vi "Test Sweep Mode vs Lockin_Vsg.vi"() -> ()   [LabVIEW 2019]
uses:
  src/Instrument.DAQ/Typedefs/Sweep.Configuration--Cluster.ctl
  src/Instrument.DAQ/Typedefs/Sweep.Channel--Cluster--Array.ctl
  src/Instrument.DAQ/Typedefs/Sweep.Channel--Cluster.ctl
  src/Instrument.DAQ/Typedefs/Sweep.Pattern--Enum.ctl
  src/Instrument.DAQ/Instrument.DAQ.lvclass
  <vilib>/measure/NI_MAPro.lvlib
  src/Instrument.Lockin/Instrument.Lockin.lvclass
  <vilib>/measure/maresamp.llb/Resample Waveform (single shot).vi
panel:
  in  "filename":string="100ms"
  in  "path":path=path "C:/user/patrick/hg/levy_inst_lockin/Tests/Test Sweep Mode/Test3"
  in  "OK":bool
  out "Sweep Mode (s)":u32=12
  out "LockinVsg (s)":u32=53
  in  "Configure Sweep":T1 {"Channels"."Table" format="%#_1f"; "Channels"."Channel" min=1 max=128; "Channels"."Start" format="%#_6p"; "Channels"."End" format="%#_6p"}
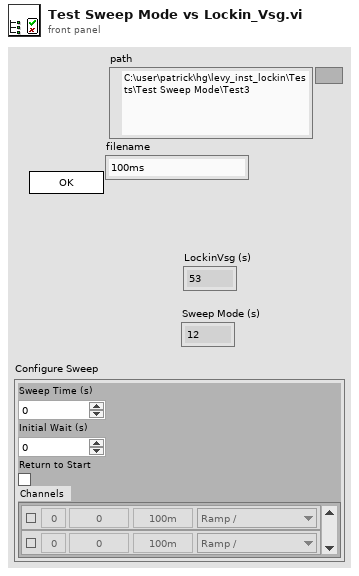
[diagram p1: front panel]
types:
  T1 = typedef "Instrument.Lockin.lvlib/Instrument.DAQ.lvclass/Sweep.Configuration--Cluster.ctl" = cluster{"Sweep Time (s)":dbl, "Initial Wait (s)":dbl, "Return to Start":bool, "Channels":T2}
  T2 = typedef "Instrument.Lockin.lvlib/Instrument.DAQ.lvclass/Sweep.Channel--Cluster--Array.ctl" = T3[]
  T3 = typedef "Instrument.Lockin.lvlib/Instrument.DAQ.lvclass/Sweep.Channel--Cluster.ctl" = cluster{"Enable?":bool, "Channel":u16, "Start":dbl, "End":dbl, "Pattern":T4, "Table":dbl[]}
  T4 = typedef "Instrument.Lockin.lvlib/Instrument.DAQ.lvclass/Sweep.Pattern--Enum.ctl" = enum16{"Ramp /", "Ramp /\\", "Smooth Ramp _/", "Smooth Ramp _/\\_", "Table"}
  T5 = enum32{"Invalid", "Standard", "Closed", "Hidden", "Minimized", "Maximized"}
  T6 = enum32{"invalid app kind", "Development System", "Run Time System", "Student Edition", "Embedded LabVIEW", "Evaluation", "Custom"}
  T7 = cluster{"Core":cluster{"Current VI Reference":refnum<vi>, "Close Panel on Exit?":bool}, "WFMs":waveform(dbl)[]}
  T8 = cluster{"Current VI Reference":refnum<vi>, "Close Panel on Exit?":bool}
  T9 = cluster{"Waveform Graph":dbl[], cluster{"key":string, "value":dbl}[]}
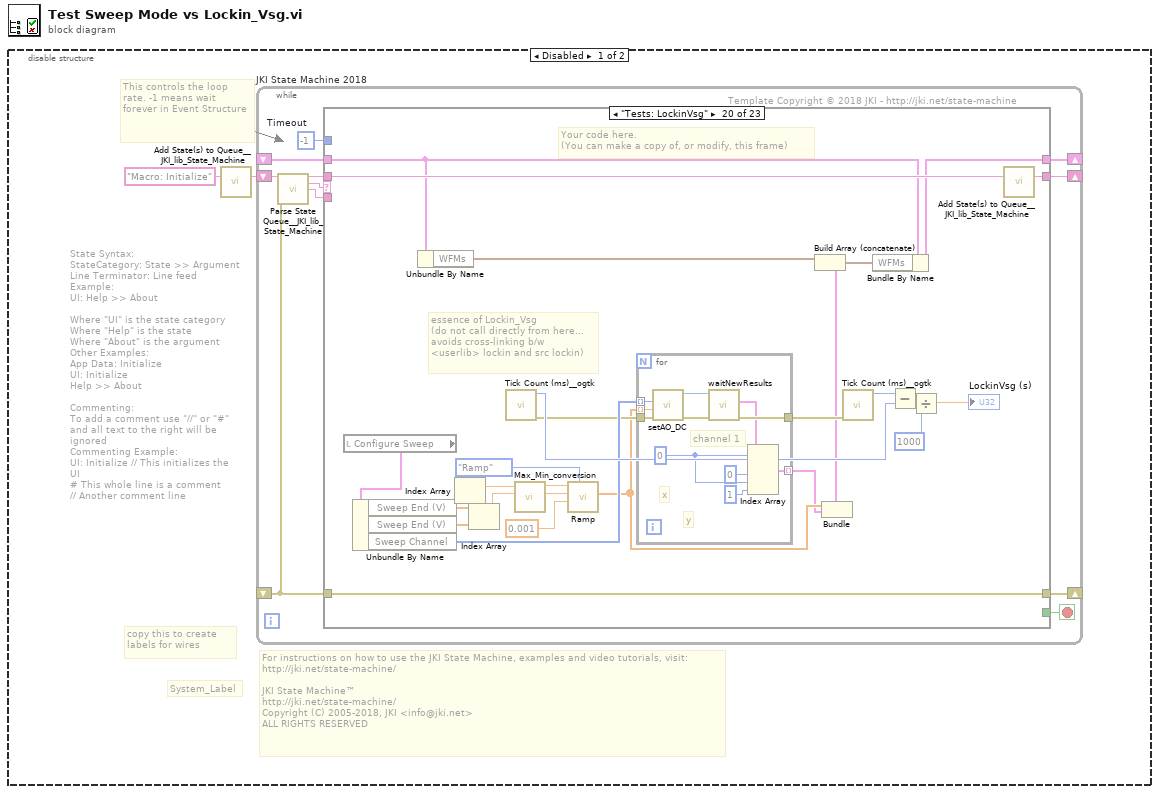
[diagram p0: block diagram]
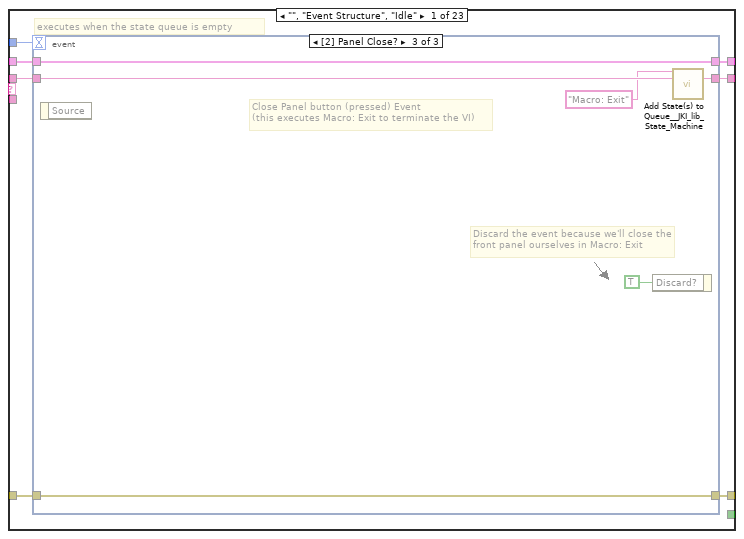
[diagram p2: hidden frame]
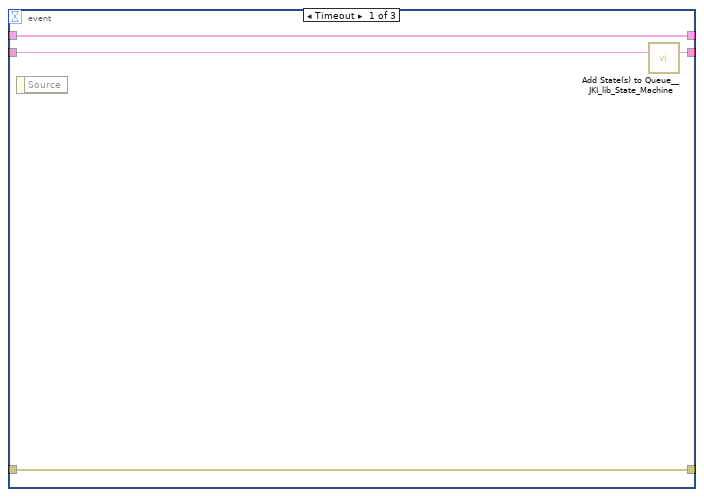
[diagram p3: hidden frame]
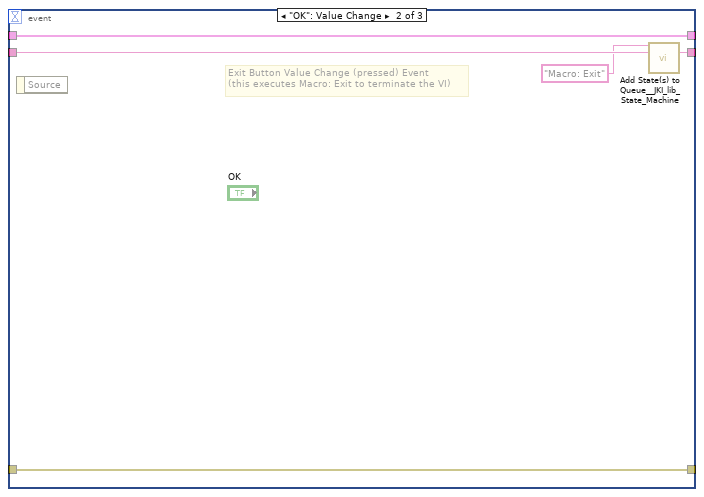
[diagram p4: hidden frame]
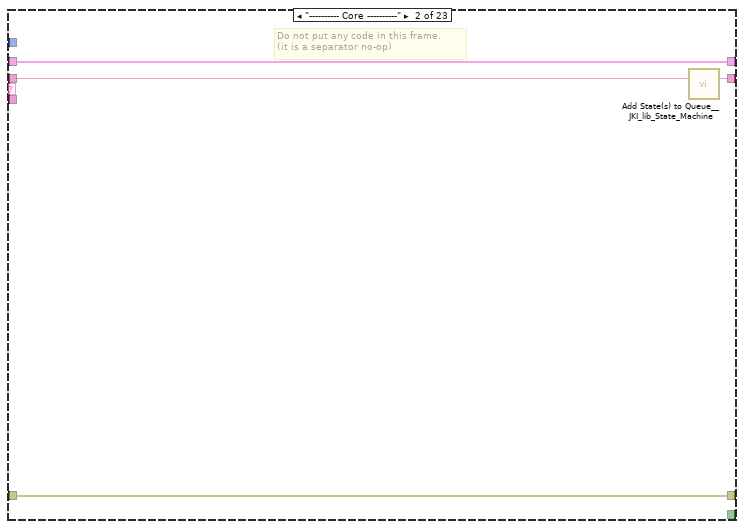
[diagram p5: hidden frame]
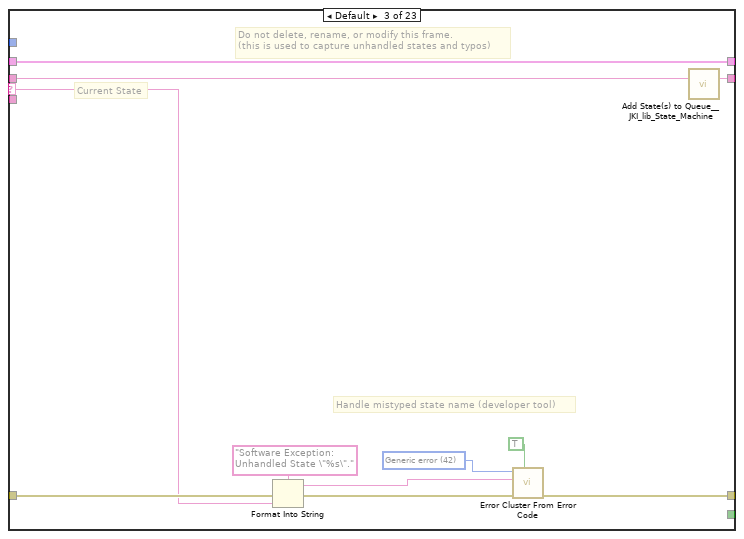
[diagram p6: hidden frame]
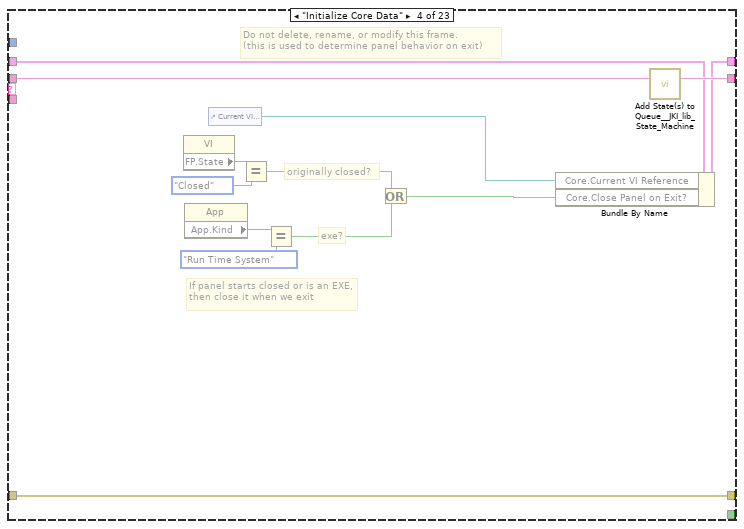
[diagram p7: hidden frame]
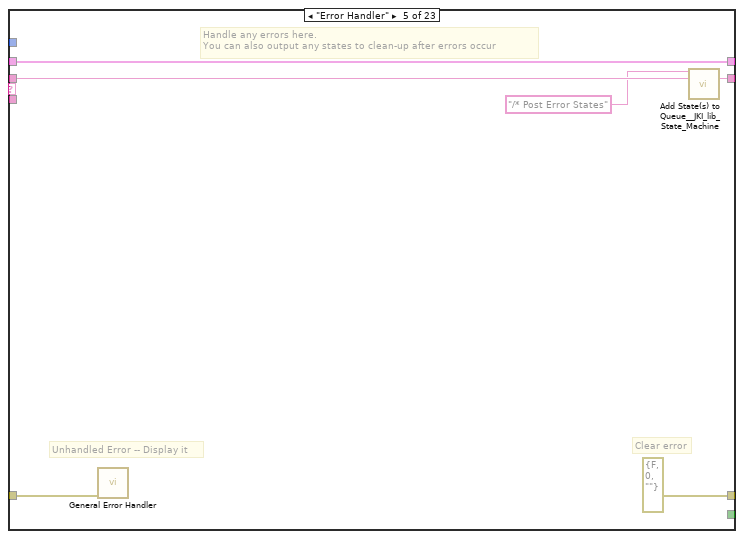
[diagram p8: hidden frame]
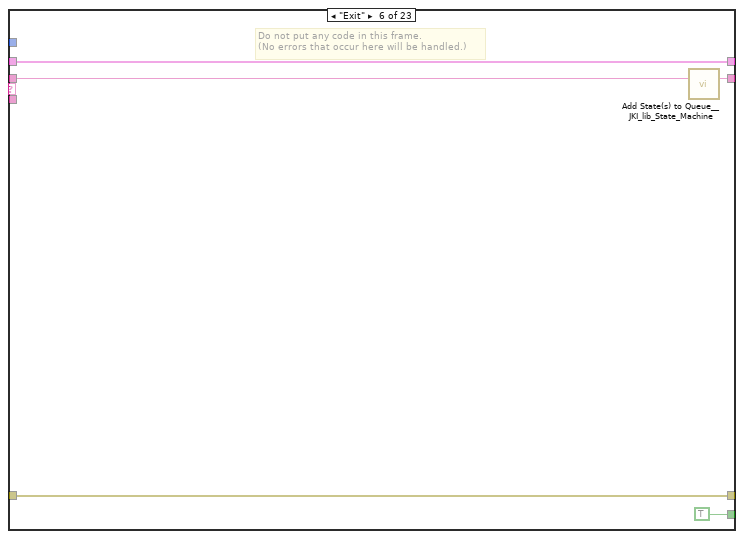
[diagram p9: hidden frame]
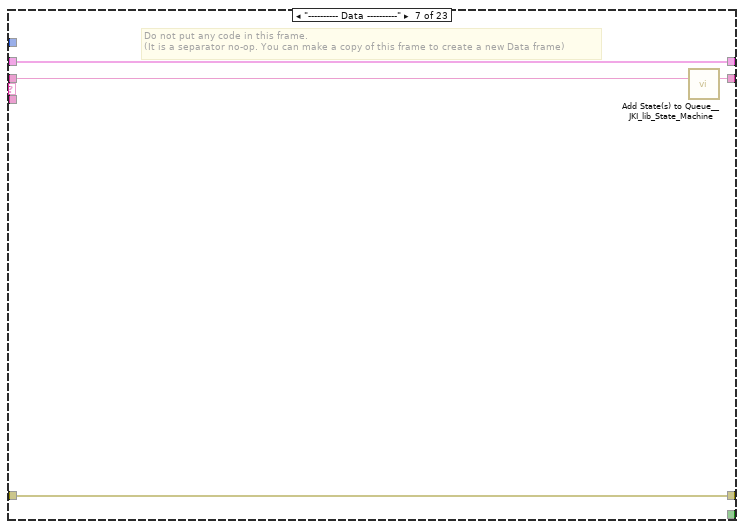
[diagram p10: hidden frame]
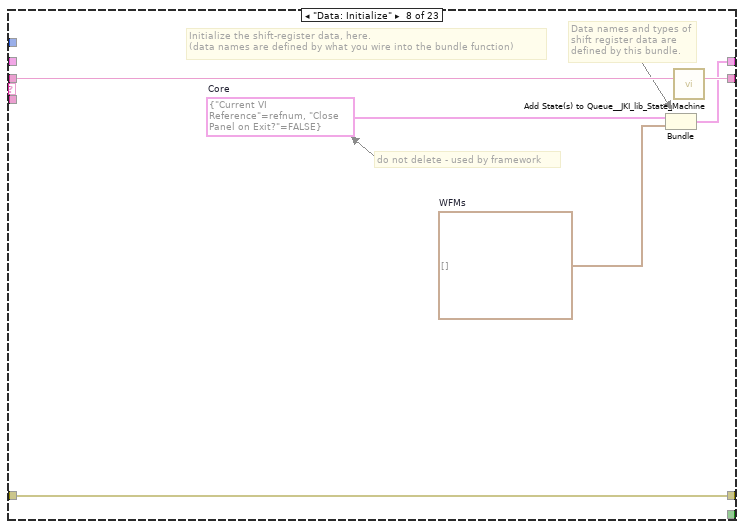
[diagram p11: hidden frame]
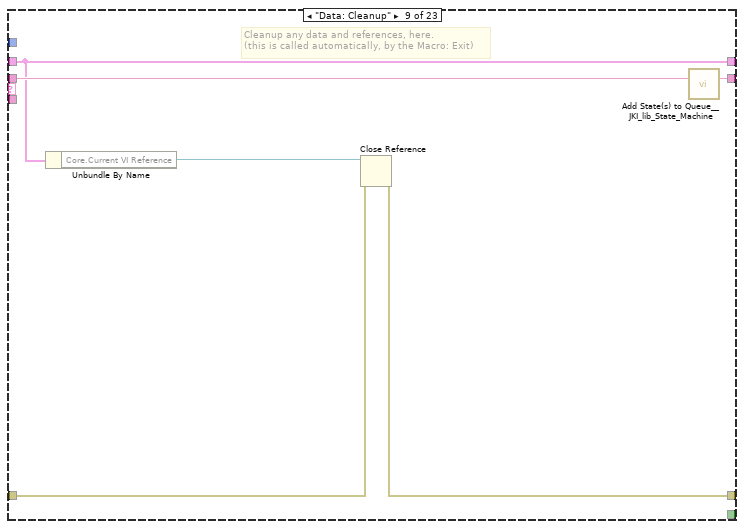
[diagram p12: hidden frame]
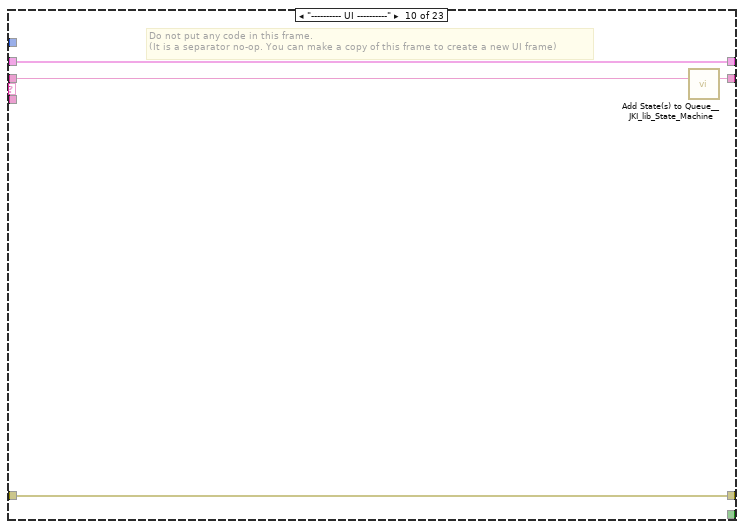
[diagram p13: hidden frame]
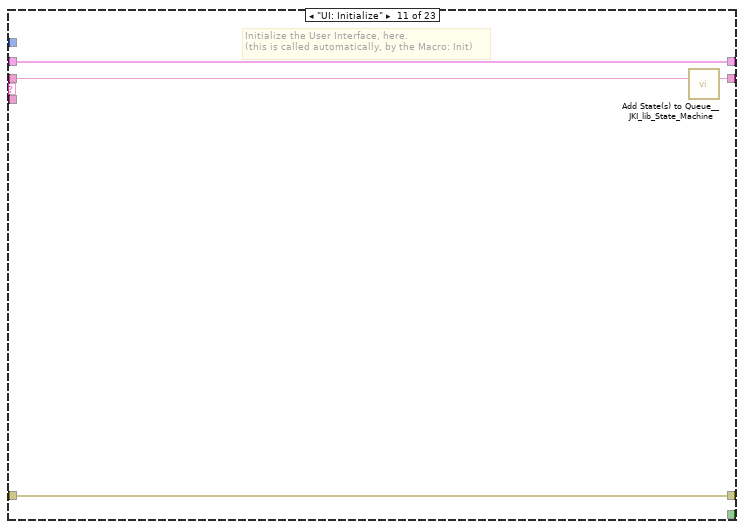
[diagram p14: hidden frame]
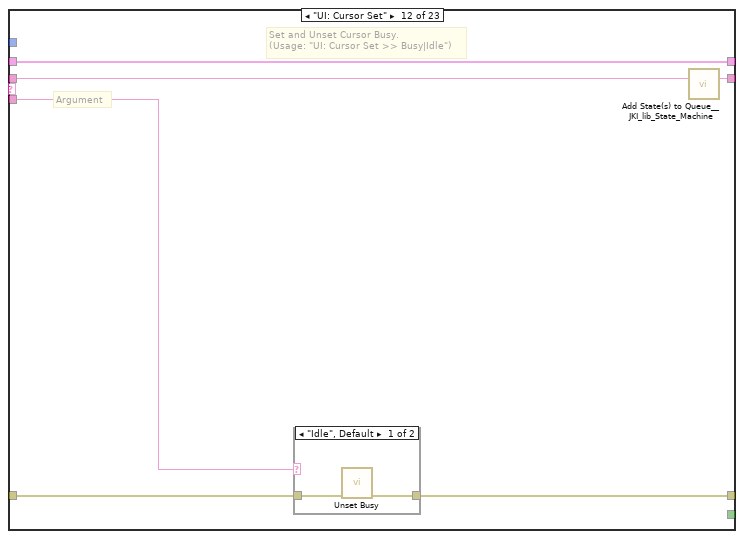
[diagram p15: hidden frame]
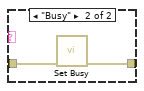
[diagram p16: hidden frame]
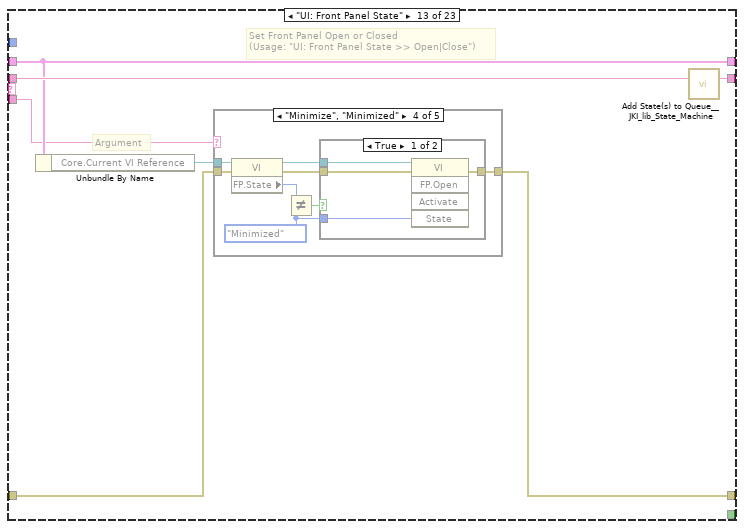
[diagram p17: hidden frame]
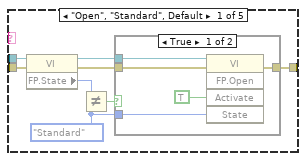
[diagram p18: hidden frame]
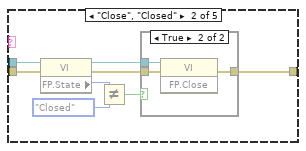
[diagram p20: hidden frame]
diagram:
  n1 = disable-structure shown="Disabled" {
    frame Disabled {
      # "For instructions on how to use the JKI State Machine, examples and video tutorials, visit:\nhttp://jki.net/state-machine/\n\nJKI State Machine™\nhttp://jki.net/state-machine/\nCopyright (C) 2005-2018, JKI <info@jki.net>\nALL RIGHTS RESERVED"
      # "State Syntax:\nStateCategory: State >> Argument\nLine Terminator: Line feed\nExample:\nUI: Help >> About\n\nWhere \"UI\" is the state category\nWhere \"Help\" is the state\nWhere \"About\" is the argument\nOther Examples:\nApp Data: Initialize\nUI: Initialize\nHelp >> About\n\nCommenting:\nTo add a comment use \"//\" or \"#\" and all text to the right will be ignored\nCommenting Example:\nUI: Initialize // This initializes the UI\n# This whole line is a comment\n// Another comment line"
      # "copy this to create labels for wires"
      # "This controls the loop rate. -1 means wait forever in Event Structure"
      # "System_Label"
      n2 = call <vilib>:"Add State(s) to Queue__JKI_lib_State_Machine.vi"("State(s) in (\"\")"="Macro: Initialize") -> ("States Out"=w2:string)  [unwired: 14 in]
      n3 = while "JKI State Machine 2018" {
        shift-right: [w6] -> _
        shift-left: _ -> [w5]
        shift-right: [w9] -> _
        shift-left: _ -> [w3]
        shift-right: [w8] -> _
        shift-left: w2 -> [w10]
        stop <- w7 stop-if-true
        w4 = -1  # Timeout
        # "Template Copyright © 2018 JKI - http://jki.net/state-machine"
        n4 = call <vilib>:"Parse State Queue__JKI_lib_State_Machine.vi"("State Queue"=w10, "Error In (no error)"=w3) -> ("Remaining States"=w12:string, "Current State"=w13:string, "Arguments"=w11:string)  [unwired: 11 in]
        n5 = case shown="\"Tests: LockinVsg\"" w13 {
          selector: w13 -> [_ _ w40 _ _ _ _ _ _ _ _ _ _ _ _ _ _ _ _ _ _ _ _]
          tunnel: w12 -> [w20 w39 w44 w63 w69 w74 w78 w84 w90 w94 w98 w104 w115 w184 w189 w194 w204 w208 w234 w261 w282 w305 w332]
          tunnel: w11 -> [_ _ _ _ _ _ _ _ _ _ _ w99 w109 _ _ _ _ _ w213 _ _ _ _]
          tunnel: w5 -> [w18 w36 w42 w56 w66 w72 w75 _ w85 w91 w96 w102 w111 w181 w186 w191 w201 w205 w218 w253 w275 w298 w329]
          tunnel: [w17 w37 w46 w60 errorcluster {"status"=FALSE, "code"=0, "source"=""} ("error out") w71 w76 w80 w86 w92 w95 w100 w112 w182 w187 w192 w202 w206 w219 w259 w280 w302 w330] -> w9
          tunnel: w3 -> [w16 w37 w45 w60 w65 w71 w76 w80 w87 w92 w95 w101 w113 w182 w187 w192 w202 w206 w220 w259 w280 w303 w330]
          tunnel: [w19 w38 w43 w62 w68 w73 w77 w83 w89 w93 w97 w103 w114 w183 w188 w193 w203 w207 w233 w260 w281 w304 w331] -> w8
          tunnel: [_ _ _ _ _ TRUE _ _ _ _ _ _ _ _ _ _ _ _ _ _ _ _ _] -> w7
          tunnel: [w15 w36 w42 w61 w66 w72 w75 w82 w85 w91 w96 w102 w111 w181 w186 w191 w201 w205 w217 w252 w274 w297 w329] -> w6
          tunnel: w4 -> [w14 _ _ _ _ _ _ _ _ _ _ _ _ _ _ _ _ _ _ _ _ _ _]
          frame "", "Event Structure", "Idle" {
            # "executes when the state queue is empty"
            n6 = event shown="[2] Panel Close?" {
              selector: _ -> [_ _ _]
              dyn-events: _ -> [_ _ _]
              timeout: w14 -> [_ _ _]
              tunnel: w20 -> [w24 w29 w35]
              tunnel: [w23 w28 w34] -> w19
              tunnel: w18 -> [w21 w26 w32]
              tunnel: [w22 w27 w33] -> w17
              tunnel: w16 -> [w22 w27 w33]
              tunnel: [w21 w26 w32] -> w15
              event Timeout {
                n7 = event-data() -> ()  [unwired: 1 in, 1 out]
                n8 = call <vilib>:"Add State(s) to Queue__JKI_lib_State_Machine.vi"("State(s) in (\"\")"=w24) -> ("States Out"=w23:string)  [unwired: 14 in]
              }
              event "OK": Value Change {
                # "Exit Button Value Change (pressed) Event\n(this executes Macro: Exit to terminate the VI)"
                n9 = event-data() -> ()  [unwired: 1 in, 1 out]
                n10 = call <vilib>:"Add State(s) to Queue__JKI_lib_State_Machine.vi"("State(s) in Front (\"\")"="Macro: Exit", "State(s) in (\"\")"=w29) -> ("States Out"=w28:string)  [unwired: 13 in]
              }
              event Panel Close? {
                # "Discard the event because we'll close the front panel ourselves in Macro: Exit"
                # "Close Panel button (pressed) Event\n(this executes Macro: Exit to terminate the VI)"
                n11 = event-data() -> ()  [unwired: 1 in, 1 out]
                n12 = event-data("Discard?"=TRUE) -> ()  [unwired: 1 in, 1 out]
                n13 = call <vilib>:"Add State(s) to Queue__JKI_lib_State_Machine.vi"("State(s) in Front (\"\")"="Macro: Exit", "State(s) in (\"\")"=w35) -> ("States Out"=w34:string)  [unwired: 13 in]
              }
            }
          }
          frame "---------- Core ----------" {
            # "Do not put any code in this frame.\n(it is a separator no-op)"
            n14 = call <vilib>:"Add State(s) to Queue__JKI_lib_State_Machine.vi"("State(s) in (\"\")"=w39) -> ("States Out"=w38:string)  [unwired: 14 in]
          }
          frame Default {
            w49 = 42 items=["No error", "Argument error", "Memory is full", "Out of zone", "End of file", "File already open", "Generic file I/O error", "File not found", "File permission error", "Disk is full", "Duplicate path", "Too many files open", "System feature not enabled", "Resource file not found", "Cannot add resource", "Resource not found", "Image not found", "Image memory error", "Pen does not exist", "Config type invalid", "Config token not found", "Config parse error", "Config memory error", "Bad external code format", "Bad external code offset", "External code not present", "Null window", "Destroy window error", "Null menu", "Print aborted", "Bad print record", "Print driver error", "Windows error during printing", "Memory error during printing", "Print dialog error", "Generic print error", "Invalid device refnum", "Device not found", "Device parameter error", "Device unit error", "Cannot open device", "Device call aborted", "Generic error", "Cancelled by user", "Object ID too low", "Object ID too high", "Object not in heap", "Unknown heap", "Unknown object (invalid DefProc)", "Unknown object (DefProc not in table)", "Message out of range", "Invalid (null) method", "Unknown message", "Manager call not supported", "Bad address", "Network operation in progress", "Network operation timed out", "Connection is busy", "Network attribute not supported", "Network error", "Address in use", "System out of memory", "Connection aborted", "Connection refused", "Not connected", "Already connected", "Connection closed", "Initialization error (interapplication manager)", "Bad occurrence", "Wait on unbound occurrence handler", "Occurrence queue overflow", "Datalog type conflict", "Unused", "Unrecognized type (interapplication manager)", "Memory corrupt", "Failed to make temporary DLL", "Old CIN version", "Drag socket not found", "Failed to load drop-object", "Failed to register OLE object", "Failed to release OLE object", "Format specifier type mismatch", "Unknown format specifier", "Too few format specifiers", "Too many format specifiers", "Scan failed", "Newer CIN version", "Error converting to variant", "Runtime menu error", "Password tampered", "Variant attribute not found", "Incompatible variant data type", "Event data is not available", "Event Store is not present", "Occurrence is not found", "Event Queue is not created", "Event info is not available", "Refnum passed is NULL", "Error retrieving Class GUID", "Error retrieving CoClass GUID", "Error retrieving TypeLib GUID.", "Bad built application magic bytes.", "Specific driver is different from the specific driver associated with the Logical Name.", "There is no session opened to the class driver.", "Max Error", "MAX - Error with config objects", "MAX - Error loading configuration", "MAX - Group not supported"]
            # "Current State"
            # "Do not delete, rename, or modify this frame.\n(this is used to capture unhandled states and typos)"
            # "Handle mistyped state name (developer tool)"
            n15 = Format Into String(format string="Software Exception: Unhandled State \"%s\"." ("message"), error in=w45, w40) -> (resulting string=w48:string, error out=w47:errorcluster)  [unwired: 1 in]
            n16 = call <vilib>:"Error Cluster From Error Code.vi"("show call chain? (False)"=TRUE, "error in (no error)"=w47, "error message (\"\")"=w48, "error code (0)"=w49) -> ("error out"=w46:errorcluster)  [unwired: 5 in]
            n17 = call <vilib>:"Add State(s) to Queue__JKI_lib_State_Machine.vi"("State(s) in (\"\")"=w44) -> ("States Out"=w43:string)  [unwired: 14 in]
          }
          frame "Initialize Core Data" {
            # "Do not delete, rename, or modify this frame.\n(this is used to determine panel behavior on exit)"
            # "originally closed?"
            # "exe?"
            # "If panel starts closed or is an EXE, then close it when we exit"
            n18 = property class="VI"() -> ("FP.State"=w53:T5)  [unwired: 2 in, 2 out]
            n19 = property class="App"() -> ("App.Kind"=w59:T6)  [unwired: 2 in, 2 out]
            n20 = control-ref of="Current VI Reference"() -> (w54:refnum<vi>)
            n21 = Equal?(x=w53, y=T5."Closed" ("Front Panel Window:State")) -> (x = y?=w51:bool)
            n22 = Equal?(x=w59, y=T6."Run Time System" ("Application:Kind")) -> (x = y?=w57:bool)
            n23 = Or(x=w51, y=w57) -> (x .or. y?=w55:bool)
            n24 = Bundle By Name(cluster=w56, "Core.Current VI Reference"=w54, "Core.Close Panel on Exit?"=w55) -> (w61:T7)
            n25 = call <vilib>:"Add State(s) to Queue__JKI_lib_State_Machine.vi"("State(s) in (\"\")"=w63) -> ("States Out"=w62:string)  [unwired: 14 in]
          }
          frame "Error Handler" {
            # "Unhandled Error -- Display it"
            # "Handle any errors here.\nYou can also output any states to clean-up after errors occur"
            # "Clear error"
            n26 = call <vilib>:"General Error Handler.vi"("error in (no error)"=w65) -> ()  [unwired: 10 in, 5 out]
            n27 = call <vilib>:"Add State(s) to Queue__JKI_lib_State_Machine.vi"("State(s) in Front (\"\")"="/* Post Error States", "State(s) in (\"\")"=w69) -> ("States Out"=w68:string)  [unwired: 13 in]
          }
          frame "Exit" {
            # "Do not put any code in this frame.\n(No errors that occur here will be handled.)"
            n28 = call <vilib>:"Add State(s) to Queue__JKI_lib_State_Machine.vi"("State(s) in (\"\")"=w74) -> ("States Out"=w73:string)  [unwired: 14 in]
          }
          frame "---------- Data ----------" {
            # "Do not put any code in this frame.\n(It is a separator no-op. You can make a copy of this frame to create a new Data frame)"
            n29 = call <vilib>:"Add State(s) to Queue__JKI_lib_State_Machine.vi"("State(s) in (\"\")"=w78) -> ("States Out"=w77:string)  [unwired: 14 in]
          }
          frame "Data: Initialize" {
            w79 = waveform(dbl)[] []  # WFMs
            w81 = T8 {"Current VI Reference"=refnum, "Close Panel on Exit?"=FALSE}  # Core
            # "do not delete - used by framework"
            # "Data names and types of shift register data are defined by this bundle."
            # "Initialize the shift-register data, here.\n(data names are defined by what you wire into the bundle function)"
            n30 = Bundle("Core"=w81, "WFMs"=w79) -> (w82:T7)  [unwired: 1 in]
            n31 = call <vilib>:"Add State(s) to Queue__JKI_lib_State_Machine.vi"("State(s) in (\"\")"=w84) -> ("States Out"=w83:string)  [unwired: 14 in]
          }
          frame "Data: Cleanup" {
            # "Cleanup any data and references, here.\n(this is called automatically, by the Macro: Exit)"
            n32 = Unbundle By Name(w85) -> ("Core.Current VI Reference"=w88:refnum<vi>)
            n33 = Close Reference(reference=w88, error in (no error)=w87) -> (error out=w86:errorcluster)
            n34 = call <vilib>:"Add State(s) to Queue__JKI_lib_State_Machine.vi"("State(s) in (\"\")"=w90) -> ("States Out"=w89:string)  [unwired: 14 in]
          }
          frame "---------- UI ----------" {
            # "Do not put any code in this frame.\n(It is a separator no-op. You can make a copy of this frame to create a new UI frame)"
            n35 = call <vilib>:"Add State(s) to Queue__JKI_lib_State_Machine.vi"("State(s) in (\"\")"=w94) -> ("States Out"=w93:string)  [unwired: 14 in]
          }
          frame "UI: Initialize" {
            # "Initialize the User Interface, here.\n(this is called automatically, by the Macro: Init)"
            n36 = call <vilib>:"Add State(s) to Queue__JKI_lib_State_Machine.vi"("State(s) in (\"\")"=w98) -> ("States Out"=w97:string)  [unwired: 14 in]
          }
          frame "UI: Cursor Set" {
            # "Argument"
            # "Set and Unset Cursor Busy.\n(Usage: \"UI: Cursor Set >> Busy|Idle\")"
            n37 = case shown="\"Idle\", Default" w99 {
              tunnel: w101 -> [w106 w108]
              tunnel: [w105 w107] -> w100
              frame "Idle", Default {
                n38 = call <vilib>:"Unset Busy.vi"("error in (no error)"=w106) -> ("error out"=w105:errorcluster)  [unwired: 10 in]
              }
              frame "Busy" {
                n39 = call <vilib>:"Set Busy.vi"("error in (no error)"=w108) -> ("error out"=w107:errorcluster)  [unwired: 9 in, 1 out]
              }
            }
            n40 = call <vilib>:"Add State(s) to Queue__JKI_lib_State_Machine.vi"("State(s) in (\"\")"=w104) -> ("States Out"=w103:string)  [unwired: 14 in]
          }
          frame "UI: Front Panel State" {
            # "Argument"
            # "Set Front Panel Open or Closed\n(Usage: \"UI: Front Panel State >> Open|Close\")"
            n41 = Unbundle By Name(w111) -> ("Core.Current VI Reference"=w110:refnum<vi>)
            n42 = case shown="\"Minimize\", \"Minimized\"" w109 {
              tunnel: w113 -> [w121 w136 w147 w160 w173]
              tunnel: [w123 w137 w149 w162 w175] -> w112
              tunnel: w110 -> [w122 w134 w148 w161 w174]
              frame "Open", "Standard", Default {
                w116 = T5."Standard" ("State")
                n43 = property class="VI"(reference=w122, error in=w121) -> (reference out=w119:refnum<vi>, error out=w120:errorcluster, "FP.State"=w118:T5)
                n44 = Not Equal?(x=w118, y=w116) -> (x != y?=w117:bool)
                n45 = case shown="True" w117 {
                  tunnel: [w127 w129] -> w123
                  tunnel: w120 -> [w126 w129]
                  tunnel: w119 -> [w125 _]
                  tunnel: w116 -> [w124 _]
                  frame True {
                    n46 = invoke class="VI" method="FP.Open"(reference=w125, error in=w126, "Activate"=TRUE, "State"=w124) -> (error out=w127:errorcluster)  [unwired: 1 in, 4 out]
                  }
                  frame False {
                  }
                }
              }
              frame "Close", "Closed" {
                n47 = property class="VI"(reference=w134, error in=w136) -> (reference out=w133:refnum<vi>, error out=w135:errorcluster, "FP.State"=w131:T5)
                n48 = Not Equal?(x=w131, y=T5."Closed" ("Front Panel Window:State")) -> (x != y?=w130:bool)
                n49 = case shown="True" w130 {
                  tunnel: [w138 w141] -> w137
                  tunnel: w135 -> [w138 w140]
                  tunnel: w133 -> [_ w139]
                  frame False {
                  }
                  frame True {
                    n50 = invoke class="VI" method="FP.Close"(reference=w139, error in=w140) -> (error out=w141:errorcluster)  [unwired: 1 in, 2 out]
                  }
                }
              }
              frame "Hidden", "Hide" {
                w142 = T5."Hidden" ("State")
                n51 = property class="VI"(reference=w148, error in=w147) -> (reference out=w145:refnum<vi>, error out=w146:errorcluster, "FP.State"=w144:T5)
                n52 = Not Equal?(x=w144, y=w142) -> (x != y?=w143:bool)
                n53 = case shown="True" w143 {
                  tunnel: [w153 w154] -> w149
                  tunnel: w146 -> [w152 w154]
                  tunnel: w145 -> [w151 _]
                  tunnel: w142 -> [w150 _]
                  frame True {
                    n54 = invoke class="VI" method="FP.Open"(reference=w151, error in=w152, "State"=w150) -> (error out=w153:errorcluster)  [unwired: 2 in, 4 out]
                  }
                  frame False {
                  }
                }
              }
              frame "Minimize", "Minimized" {
                w155 = T5."Minimized" ("State")
                n55 = property class="VI"(reference=w161, error in=w160) -> (reference out=w158:refnum<vi>, error out=w159:errorcluster, "FP.State"=w157:T5)
                n56 = Not Equal?(x=w157, y=w155) -> (x != y?=w156:bool)
                n57 = case shown="True" w156 {
                  tunnel: [w166 w167] -> w162
                  tunnel: w159 -> [w165 w167]
                  tunnel: w158 -> [w164 _]
                  tunnel: w155 -> [w163 _]
                  frame True {
                    n58 = invoke class="VI" method="FP.Open"(reference=w164, error in=w165, "State"=w163) -> (error out=w166:errorcluster)  [unwired: 2 in, 4 out]
                  }
                  frame False {
                  }
                }
              }
              frame "Maximize", "Maximized" {
                w168 = T5."Maximized" ("State")
                n59 = property class="VI"(reference=w174, error in=w173) -> (reference out=w171:refnum<vi>, error out=w172:errorcluster, "FP.State"=w170:T5)
                n60 = Not Equal?(x=w170, y=w168) -> (x != y?=w169:bool)
                n61 = case shown="True" w169 {
                  tunnel: [w179 w180] -> w175
                  tunnel: w172 -> [w178 w180]
                  tunnel: w171 -> [w177 _]
                  tunnel: w168 -> [w176 _]
                  frame True {
                    n62 = invoke class="VI" method="FP.Open"(reference=w177, error in=w178, "State"=w176) -> (error out=w179:errorcluster)  [unwired: 2 in, 4 out]
                  }
                  frame False {
                  }
                }
              }
            }
            n63 = call <vilib>:"Add State(s) to Queue__JKI_lib_State_Machine.vi"("State(s) in (\"\")"=w115) -> ("States Out"=w114:string)  [unwired: 14 in]
          }
          frame "---------- Macro ----------" {
            # "Do not put any code in this frame.\n(It is a separator no-op. You can make a copy of this frame to create a new Macro frame)"
            n64 = call <vilib>:"Add State(s) to Queue__JKI_lib_State_Machine.vi"("State(s) in (\"\")"=w184) -> ("States Out"=w183:string)  [unwired: 14 in]
          }
          frame "Macro: Initialize" {
            w185 = "Data: Initialize\nInitialize Core Data\nUI: Initialize\nUI: Front Panel State >> Open\nMacro: Test\nMacro: Exit"  # Data: Initialize Initialize Core Data UI: Initialize UI: Front Panel State >> Open Macro: Test Macro: Exit
            # "Initialization Macro\n(This is called once, when the VI starts)"
            n65 = call <vilib>:"Add State(s) to Queue__JKI_lib_State_Machine.vi"("State(s) in Front (\"\")"=w185, "State(s) in (\"\")"=w189) -> ("States Out"=w188:string)  [unwired: 13 in]
          }
          frame "Macro: Test" {
            # "Initialization Macro\n(This is called once, when the VI starts)"
            n66 = call <vilib>:"Add State(s) to Queue__JKI_lib_State_Machine.vi"("State(s) in Front (\"\")"="Tests: LockinVsg\nTests: Sweep Mode >> 60\nTests: Sweep Mode >> 30\nTests: Sweep Mode >> 15\nTests: Sweep Mode >> 10\nTests: Model\nTests: Analyze\nTests: Save", "State(s) in (\"\")"=w194) -> ("States Out"=w193:string)  [unwired: 13 in]
          }
          frame "Macro: Exit" {
            # "Exit Macro\n(This is called once, when the VI exits)"
            n67 = Unbundle By Name(w201) -> ("Core.Close Panel on Exit?"=w200:bool)
            n68 = Select(t="UI: Front Panel State >> Close", s=w200, f="") -> (s? t:f=w197:string)
            n69 = call <vilib>:"Add State(s) to Queue__JKI_lib_State_Machine.vi"("State(s) in (\"\")"=w197, "State(s) at Back (\"\")"="Data: Cleanup\nExit") -> ("States Out"=w195:string)  [unwired: 13 in]
            n70 = call <vilib>:"Add State(s) to Queue__JKI_lib_State_Machine.vi"("State(s) in Front (\"\")"=w195, "State(s) in (\"\")"=w204) -> ("States Out"=w203:string)  [unwired: 13 in]
          }
          frame "---------- Tests ----------" {
            # "Template Separator\n(You can make a copy of, or modify, this frame)"
            n71 = call <vilib>:"Add State(s) to Queue__JKI_lib_State_Machine.vi"("State(s) in (\"\")"=w208) -> ("States Out"=w207:string)  [unwired: 14 in]
          }
          frame "Tests: Sweep Mode" {
            # "Your code here.\n(You can make a copy of, or modify, this frame)"
            n72 = Scan From String(input string=w213) -> (output 1=w211:dbl)  [unwired: 4 in, 3 out]
            n73 = Bundle By Name(cluster="Configure Sweep", "Sweep Time (s)"=w211) -> (w210:T1)
            n74 = call <userlib>:"Tick Count (ms)__ogtk.vi"("error in (no error)"=w220) -> ("error out"=w228:errorcluster, "millisecond timer value"=w231:u32)  [unwired: 9 in]
            n75 = call-dynamic "Open.vi"("error in (no error)"=w228, "address"="" ("Address"), "Instrument.Lockin in"=refnum<class "Instrument.Lockin.lvclass"> refnum) -> ("error out"=w225:errorcluster, "Instrument.Lockin out"=w224:refnum<class "Instrument.Lockin.lvclass">)  [unwired: 7 in]
            n76 = call-dynamic "startSweepAndWait.vi"("error in (no error)"=w225, "time (s) [10 s]"=w210, "Instrument.Lockin in"=w224) -> ("error out"=w221:errorcluster, 2:w223)  [unwired: 6 in, 1 out]
            n77 = Unbundle By Name(w218) -> ("WFMs"=w215:waveform(dbl)[])
            n78 = Unbundle By Name(w223) -> ("Sweep_AO"=w222)
            n79 = Index Array(array=w222) -> (element=w216)  [unwired: 1 in]
            n80 = call <userlib>:"Tick Count (ms)__ogtk.vi"("error in (no error)"=w221) -> ("error out"=w219:errorcluster, "millisecond timer value"=w227:u32)  [unwired: 9 in]
            n81 = Subtract(x=w227, y=w231) -> (x-y=w226:u32)
            n82 = Build Array (concatenate)(w215, w216) -> (w214:waveform(dbl)[])
            n83 = Divide(x=w226, y=u32 1000) -> (x/y=→"Sweep Mode (s)":dbl)
            n84 = Bundle By Name(cluster=w218, "WFMs"=w214) -> (w217:T7)
            n85 = call <vilib>:"Add State(s) to Queue__JKI_lib_State_Machine.vi"("State(s) in (\"\")"=w234) -> ("States Out"=w233:string)  [unwired: 14 in]
          }
          frame "Tests: LockinVsg" {
            # "essence of Lockin_Vsg\n(do not call directly from here...\navoids cross-linking b/w\n<userlib> lockin and src lockin)"
            # "Your code here.\n(You can make a copy of, or modify, this frame)"
            n86 = local read "Configure Sweep"() -> (w247:T1)
            n87 = Unbundle By Name(w247) -> ("Sweep End (V)"=w245:dbl[], "Sweep End (V)"=w244:dbl[], "Sweep Channel"=w246:i32[])
            n88 = Unbundle By Name(w253) -> ("WFMs"=w251:waveform(dbl)[])
            n89 = Index Array(array=w245) -> (element=w236:dbl)  [unwired: 1 in]
            n90 = Index Array(array=w244) -> (element=w235:dbl)  [unwired: 1 in]
            n91 = call <userlib>:"Tick Count (ms)__ogtk.vi"() -> ("error out"=w241:errorcluster, "millisecond timer value"=w255:u32)  [unwired: 10 in]
            n92 = call <userlib>:"Max_Min_conversion.vi"("Min"=w235, "Max"=w236) -> ("offset"=w249:dbl, "Amplitude"=w248:dbl)  [unwired: 8 in]
            n93 = call <userlib>:"Ramp.vi"("function (ramp)"=enum16{"Ramp", "Triangle", "Sine"}."Ramp", "step size"=0.001, "offset"=w249, "amplitude"=w248) -> ("Waveform Graph"=w239:dbl[])  [unwired: 5 in, 2 out]
            n94 = for {
              tunnel: w246 -> [w270] mode=indexing
              tunnel: w241 -> [w269]
              tunnel: [w268] -> w240
              tunnel: w239 -> [w267] mode=indexing
              tunnel: [w262] -> w238 mode=indexing
              w263 = 0 ("disabled index (row)")
              # "y"
              # "x"
              # "channel 1"
              n95 = call-dynamic "setAO_DC.vi"("error in (no error)"=w269, "DC (V)"=w267, "AO Channel"=w270) -> ("error out"=w272:errorcluster, "Instrument.Lockin out"=w271:refnum<class "Instrument.Lockin.lvclass">)  [unwired: 7 in]
              n96 = call-dynamic "waitNewResults.vi"("error in (no error)"=w272, "Instrument.Lockin in"=w271) -> ("error out"=w268:errorcluster, "Results (Dictionary)"=w264:cluster{"key":string, "value":dbl}[])  [unwired: 7 in, 1 out]
              n97 = Index Array(array=w264, index (row) #1=w263, index (col) #1=0 ("disabled index (col)"), index (row) #2=w263, index (col) #2=1 ("disabled index (col)")) -> (element #1=w262:cluster{"key":string, "value":dbl})  [unwired: 1 out]
            }
            n98 = Bundle("Waveform Graph"=w239, w238) -> (w237:T9)  [unwired: 1 in]
            n99 = Build Array (concatenate)(w251, w237) -> (w250:waveform(dbl)[])
            n100 = call <userlib>:"Tick Count (ms)__ogtk.vi"("error in (no error)"=w240) -> ("millisecond timer value"=w254:u32)  [unwired: 9 in, 1 out]
            n101 = Bundle By Name(cluster=w253, "WFMs"=w250) -> (w252:T7)
            n102 = Subtract(x=w254, y=w255) -> (x-y=w256:u32)
            n103 = Divide(x=w256, y=u32 1000) -> (x/y=→"LockinVsg (s)":dbl)
            n104 = call <vilib>:"Add State(s) to Queue__JKI_lib_State_Machine.vi"("State(s) in (\"\")"=w261) -> ("States Out"=w260:string)  [unwired: 14 in]
          }
          frame "Tests: Model" {
            # "Template Separator\n(You can make a copy of, or modify, this frame)"
            n105 = Unbundle By Name(w275) -> ("WFMs"=w277:waveform(dbl)[])
            n106 = while {
              tunnel: [w287] -> w273 mode=indexing
              i -> [w286]
              stop <- w288 stop-if-true
              n107 = call <userlib>:"Ramp_SubVI.vi"("index"=w286, "step"=0.001, "end"=0.1, "start"=0.0) -> ("Stop?"=w288:bool, "Numeric"=w287:dbl)  [unwired: 1 in]
            }
            n108 = for {
              tunnel: w273 -> [w292] mode=indexing
              tunnel: [w290] -> w279 mode=indexing
              n109 = call "Waveguide Model.vi"("Vs (V)"=0.01 ("Vsg (V)"), "Vsg (V)"=w292) -> ("I[Vsg] (A)"=w291:dbl)  [unwired: 1 out]
              n110 = Multiply(x=50000.0 ("Vsg (V)"), y=w291) -> (x*y=w290:dbl)
            }
            n111 = Bundle(w273, w279) -> (w278:cluster{dbl[], dbl[]})  [unwired: 1 in]
            n112 = Build Array (concatenate)(w277, w278) -> (w276:waveform(dbl)[])
            n113 = Bundle By Name(cluster=w275, "WFMs"=w276) -> (w274:T7)
            n114 = call <vilib>:"Add State(s) to Queue__JKI_lib_State_Machine.vi"("State(s) in (\"\")"=w282) -> ("States Out"=w281:string)  [unwired: 14 in]
          }
          frame "Tests: Analyze" {
            # "Template Separator\n(You can make a copy of, or modify, this frame)"
            n115 = Unbundle By Name(w298) -> ("WFMs"=w296:waveform(dbl)[])
            n116 = for {
              tunnel: w296 -> [w320] mode=indexing
              tunnel: w303 -> [w318]
              tunnel: [w317] -> w302
              tunnel: [w316] -> w301 mode=indexing
              n117 = call-poly <vilib>:"Resample Waveforms (single shot).vi"("waveform in"=w320, "dt"=0.001, "t0"=0.0 ("dt"), "error in (no error)"=w318) -> (6:w316, "error out"=w317:errorcluster)  [unwired: 7 in, 3 out]
            }
            n118 = Array Size(array=w301) -> (size(s)=w300:i32)
            n119 = Decrement(x=w300) -> (x-1=w299:i32)
            n120 = for {
              N: w299 -> [w306]
              tunnel: w301 -> [w313] mode=indexing
              tunnel: w301 -> [w314]
              tunnel: [w308] -> w295 mode=indexing
              n121 = Unbundle(w313) -> (w309, w310)
              n122 = Index Array(array=w314, index (row)=w306) -> (element=w312)  [unwired: 1 in]
              n123 = Unbundle(w312) -> (w311)  [unwired: 1 out]
              n124 = Subtract(x=w311, y=w310) -> (x-y=w307:dbl)
              n125 = Bundle(w309, w307) -> (w308:cluster{void, dbl})  [unwired: 1 in]
            }
            n126 = Build Array (concatenate)(w296, w295) -> (w294:waveform(dbl)[])
            n127 = Bundle By Name(cluster=w298, "WFMs"=w294) -> (w297:T7)
            n128 = call <vilib>:"Add State(s) to Queue__JKI_lib_State_Machine.vi"("State(s) in (\"\")"=w305) -> ("States Out"=w304:string)  [unwired: 14 in]
          }
          frame "Tests: Save" {
            # "Template Separator\n(You can make a copy of, or modify, this frame)"
            n129 = Unbundle By Name(w329) -> ("WFMs"=w328:waveform(dbl)[])
            n130 = Build Array (concatenate)(string[] ["Lockin_Vsg", "Sweep Mode 60", "Sweep Mode 30", "Sweep Mode 15", "Sweep Mode 10", "Model"] ("wavenames"), string[] ["Model - Lockin_Vsg", "Model - Sweep Mode 60", "Model - Sweep Mode 30", "Model - Sweep Mode 15", "Model - Sweep Mode 10"] ("wavenames")) -> (w322:string[])
            n131 = disable-structure shown="Disabled" {
              disable-tunnel: w328 -> [w340 _]
              disable-tunnel: "filename" -> [w338 _]
              disable-tunnel: string[] ["V\\Bsg\\M (V)", "X lockin (arb)"] ("X,Y Labels") -> [w336 _]
              disable-tunnel: i32[] [0, 0] ("X,Y Log") -> [w335 _]
              disable-tunnel: w322 -> [w334 _]
              disable-tunnel: "path" -> [w333 _]
              frame Disabled {
                n132 = call <userlib>:"Format Path and Filename.vi"("filename"=w338, "path"=w333) -> ("path"=w339:path)  [unwired: 7 in, 2 out]
                n133 = call <userlib>:"XY Plot Commands.vi"("X,Y Log"=w335, "Plot labels"=w334, "X,Y Labels"=w336, "wavenames"=w334) -> ("result string"=w337:string)  [unwired: 2 in]
                n134 = call <userlib>:"LV to ITX 2.2 XY.vi"("Commands"=w337, "filename"=w339, "wavenames"=w334, "XY Array"=w340) -> ()  [unwired: 7 in, 1 out]
              }
              frame Enabled {
              }
            }
            n135 = call <vilib>:"Add State(s) to Queue__JKI_lib_State_Machine.vi"("State(s) in (\"\")"=w332) -> ("States Out"=w331:string)  [unwired: 14 in]
          }
        }
      }
    }
    frame Enabled {
    }
  }
